vi "Kaelus PIM Config Test.vi"(7 "Str Refnum":refnum<vi>, 8 "error in (no error)":errorcluster, 11 "PIM Configuration":T1={"host IP (localhost)"="localhost", "host Port"=3388, "Model"="", "Serial Number(s)"="", "Calibration Date"=3388.0, "Dual Port?"=FALSE, "DeviceNames"=[], "Parameters"={"TX1start"=0.0, "TX1stop"=0.0, "TX1pmax"=0.0, "TX2start"=0.0, "TX2stop"=0.0, "TX2pmax"=0.0, "RXstart"=0.0, "RXstop"=0.0}, "Interface"=enum."PIM Web Engine"} {"Calibration Date" format="%.2f"; "Parameters"."TX2pmax" format="%.1f"; "Parameters"."TX1pmax" format="%.1f"; "Parameters"."RXstop" format="%.1f"; "Parameters"."RXstart" format="%.1f"; "Parameters"."TX2stop" format="%.1f"; "Parameters"."TX2start" format="%.1f"; "Parameters"."TX1stop" format="%.1f"; "Parameters"."TX1start" format="%.1f"}) -> (0 "error out":errorcluster, 2 "CAL Date (seconds)":dbl, 3 "Serial Number(s)":string)   [LabVIEW 2011]
uses:
  PIM Configuration.ctl
  PIM Interface Language.ctl
  TypeDefs/PIMHW Connection CMDS.ctl
  <userlib>/_OpenG.lib/array/array.llb/Remove Duplicates from 1D Array (String)__ogtk.vi
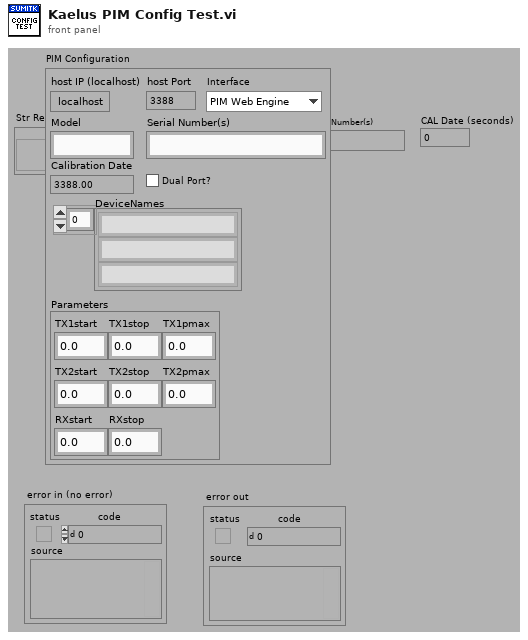
[diagram p1: front panel]
types:
  T1 = typedef "PIM Configuration.ctl" = cluster{"host IP (localhost)":string, "host Port":u16, "Model":string, "Serial Number(s)":string, "Calibration Date":dbl, "Dual Port?":bool, "DeviceNames":string[], "Parameters":cluster{"TX1start":dbl, "TX1stop":dbl, "TX1pmax":dbl, "TX2start":dbl, "TX2stop":dbl, "TX2pmax":dbl, "RXstart":dbl, "RXstop":dbl}, "Interface":T2}
  T2 = typedef "PIM Interface Language.ctl" = enum16{"PIM Web Engine", "PIM HW Engine"}
  T3 = typedef "PIMHW Connection CMDS.ctl" = enum16{"CONNECT", "DISCONNECT", "KEEP_ALIVE"}
  T4 = typedef "Test Set Definition.ctl" = cluster{"General":cluster{"ID":u32, "Model":string, "Dual Port?":bool, "Options String":string, "Options":cluster{"E":bool, "K":bool, "H":bool, "W":bool, "F":bool}, "Cal File":path}, "Receiver":cluster{"Fstart, MHz":dbl, "Fstop MHz":dbl, "Fstep MHz":dbl, "IF, MHz":dbl}, "RX Band":cluster{"Fstart, MHz":dbl, "Fstop MHz":dbl}, "TX 1":cluster{"Fstart, MHz":dbl, "Fstop MHz":dbl, "Pmax, dBm":dbl, "Pstep, dB":dbl}, "TX 2":cluster{"Fstart, MHz":dbl, "Fstop MHz":dbl, "Pmax, dBm":dbl, "Pstep, dB":dbl}, "Low-side?":bool}
  T5 = cluster{"CalVersion":u8, "CalDate":string, "CalSN":string}
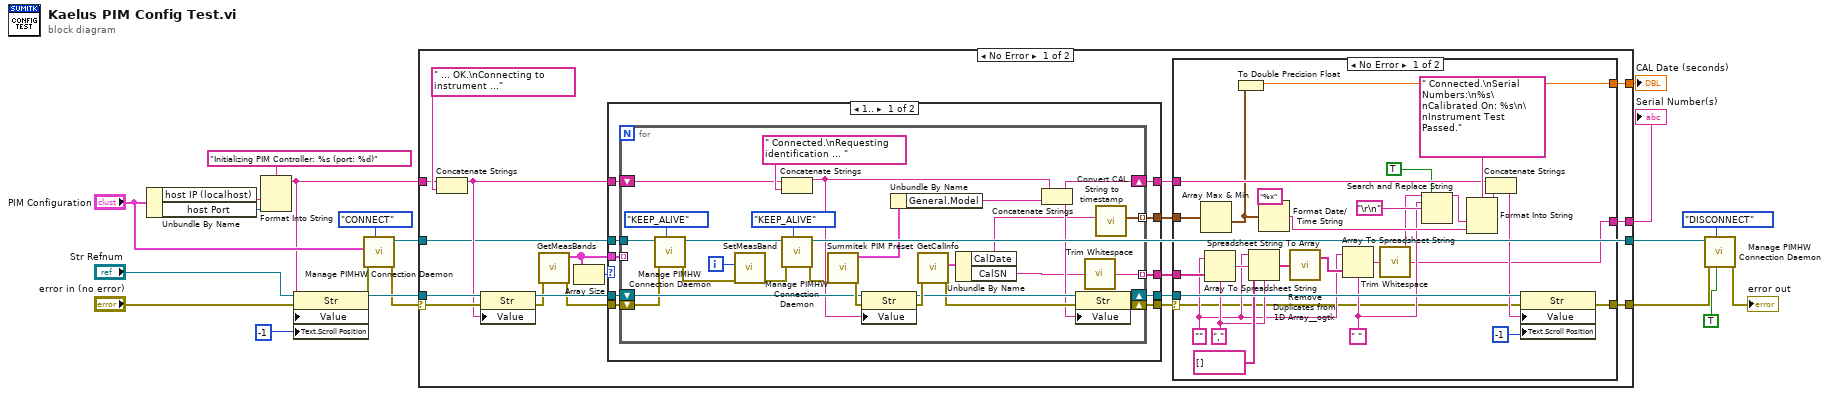
[diagram p0: block diagram]
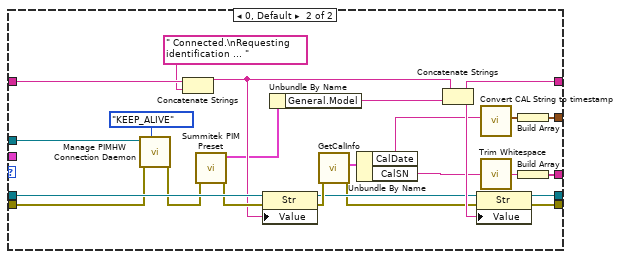
[diagram p2: hidden frame]
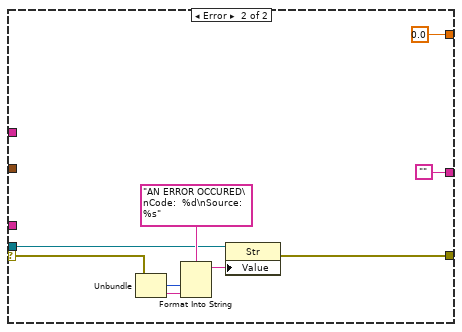
[diagram p3: hidden frame]
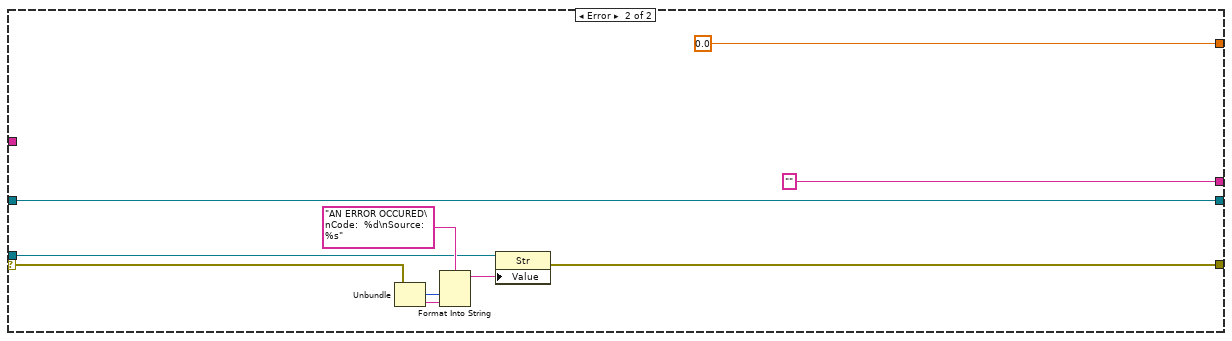
[diagram p4: hidden frame]
diagram:
  n1 = Unbundle By Name("PIM Configuration") -> ("host IP (localhost)"=w19:string, "host Port"=w18:u16)
  n2 = Format Into String(format string="Initializing PIM Controller: %s (port: %d)", w19, w18) -> (resulting string=w12:string)  [unwired: 2 in, 1 out]
  n3 = property class="Str"(reference="Str Refnum", error in="error in (no error)", "Value"=w12, "Text.Scroll Position"=-1) -> (reference out=w11:refnum<vi>, error out=w4:errorcluster)
  n4 = call "Manage PIMHW Connection Daemon.vi"("Session Conn Cmd"=PIMHW_Connection_CMDS."CONNECT", "error in (no error)"=w4, "PIM Config (Connection only)"="PIM Configuration") -> ("error out"=w2:errorcluster, "daemon ref out"=w13:refnum<vi>)  [unwired: 2 in, 5 out]
  n5 = case shown="No Error" w2 {
    selector: w2 -> [w36 w142]
    tunnel: w13 -> [w26 w139]
    tunnel: w12 -> [w38 _]
    tunnel: w11 -> [w37 w141]
    tunnel: [w33 w140] -> w7
    tunnel: [w24 "" ("CalSN")] -> w10
    tunnel: [w26 w139] -> w5
    tunnel: [w27 0.0] -> w1
    frame No Error {
      n6 = Concatenate Strings(w38, " ... OK.\nConnecting to instrument ...") -> (w35:string)
      n7 = property class="Str"(reference=w37, error in=w36, "Value"=w35) -> (reference out=w34:refnum<vi>, error out=w30:errorcluster)
      n8 = call "GetMeasBands.vi"("error in (no error)"=w30) -> ("error out"=w29:errorcluster, "TestSets"=w22:T4[])  [unwired: 1 in, 8 out]
      n9 = Array Size(array=w22) -> (size(s)=w21:i32)
      n10 = case shown="1.." w21 {
        tunnel: w35 -> [w49 w100]
        tunnel: w34 -> [w48 w99]
        tunnel: [w47 w98] -> w32
        tunnel: [w46 w97] -> w31
        tunnel: w29 -> [w45 w81]
        tunnel: w22 -> [w44 _]
        tunnel: [w43 w79] -> w28
        tunnel: w26 -> [w42 w96]
        tunnel: [w41 w78] -> w25
        tunnel: [w40 w95] -> w23
        frame 1.. {
          n11 = for {
            shift-right: [w63] -> w46
            shift-left: w49 -> [w75]
            tunnel: [w56] -> w41 mode=indexing
            shift-right: [w67] -> w40
            shift-left: w45 -> [w53]
            shift-right: [w68] -> w47
            shift-left: w48 -> [w73]
            tunnel: w44 -> [_] mode=indexing
            tunnel: [w60] -> w43 mode=indexing
            tunnel: w42 -> [w51]
            i -> [w62]
            n12 = call "Manage PIMHW Connection Daemon.vi"("Session Conn Cmd"=PIMHW_Connection_CMDS."KEEP_ALIVE", "error in (no error)"=w53, "daemon ref"=w51) -> ("error out"=w52:errorcluster, "daemon ref out"=w50:refnum<vi>)  [unwired: 2 in, 5 out]
            n13 = call "SetMeasBand.vi"("error in (no error)"=w52, "Band Index"=w62) -> ("error out"=w58:errorcluster)  [unwired: 1 in, 8 out]
            n14 = Concatenate Strings(w75, " Connected.\nRequesting identification ... ") -> (w66:string)
            n15 = call "Manage PIMHW Connection Daemon.vi"("Session Conn Cmd"=PIMHW_Connection_CMDS."KEEP_ALIVE", "error in (no error)"=w58, "daemon ref"=w50) -> ("error out"=w57:errorcluster)  [unwired: 2 in, 6 out]
            n16 = call "Summitek PIM Preset.vi"("error in (no error)"=w57) -> ("error out"=w74:errorcluster, "TestSetDef"=w65:T4)  [unwired: 2 in, 7 out]
            n17 = property class="Str"(reference=w73, error in=w74, "Value"=w66) -> (reference out=w70:refnum<vi>, error out=w72:errorcluster)
            n18 = Unbundle By Name(w65) -> ("General.Model"=w64:string)
            n19 = call "GetCalInfo.vi"("error in (no error)"=w72) -> ("error out"=w69:errorcluster, "CalInfo"=w71:T5)  [unwired: 1 in, 8 out]
            n20 = Unbundle By Name(w71) -> ("CalDate"=w61:string, "CalSN"=w55:string)
            n21 = Concatenate Strings(w66, w64) -> (w63:string)
            n22 = property class="Str"(reference=w70, error in=w69, "Value"=w63) -> (reference out=w68:refnum<vi>, error out=w67:errorcluster)
            n23 = call <vilib>:"Trim Whitespace.vi"("string"=w55) -> ("trimmed string"=w56:string)  [unwired: 1 in]
            n24 = call "Convert CAL String to timestamp.vi"("abbreviated date string"=w61) -> ("time stamp"=w60:timestamp)  [unwired: 10 out]
          }
        }
        frame 0, Default {
          n25 = call "Manage PIMHW Connection Daemon.vi"("Session Conn Cmd"=PIMHW_Connection_CMDS."KEEP_ALIVE", "error in (no error)"=w81, "daemon ref"=w96) -> ("error out"=w83:errorcluster)  [unwired: 2 in, 6 out]
          n26 = Concatenate Strings(w100, " Connected.\nRequesting identification ... ") -> (w88:string)
          n27 = call "Summitek PIM Preset.vi"("error in (no error)"=w83) -> ("error out"=w93:errorcluster, "TestSetDef"=w87:T4)  [unwired: 2 in, 7 out]
          n28 = property class="Str"(reference=w99, error in=w93, "Value"=w88) -> (reference out=w90:refnum<vi>, error out=w92:errorcluster)
          n29 = Unbundle By Name(w87) -> ("General.Model"=w86:string)
          n30 = call "GetCalInfo.vi"("error in (no error)"=w92) -> ("error out"=w89:errorcluster, "CalInfo"=w91:T5)  [unwired: 1 in, 8 out]
          n31 = Unbundle By Name(w91) -> ("CalDate"=w85:string, "CalSN"=w82:string)
          n32 = Concatenate Strings(w88, w86) -> (w97:string)
          n33 = property class="Str"(reference=w90, error in=w89, "Value"=w97) -> (reference out=w98:refnum<vi>, error out=w95:errorcluster)
          n34 = call "Convert CAL String to timestamp.vi"("abbreviated date string"=w85) -> ("time stamp"=w80:timestamp)  [unwired: 10 out]
          n35 = call <vilib>:"Trim Whitespace.vi"("string"=w82) -> ("trimmed string"=w77:string)  [unwired: 1 in]
          n36 = Build Array(w80) -> (w79:timestamp[])
          n37 = Build Array(w77) -> (w78:string[])
        }
      }
      n38 = case shown="No Error" w23 {
        selector: w23 -> [w102 w131]
        tunnel: [w126 w130] -> w33
        tunnel: w32 -> [w123 w127]
        tunnel: w31 -> [w122 _]
        tunnel: w28 -> [w117 _]
        tunnel: [w116 0.0] -> w27
        tunnel: w25 -> [w111 _]
        tunnel: [w101 ""] -> w24
        frame No Error {
          w107 = "" ("format string")
          w109 = "," ("delimiter (Tab)")
          w105 = " " ("delimiter (Tab)")
          n39 = Array Max & Min(array=w117) -> (min value=w115:timestamp)  [unwired: 3 out]
          n40 = Array To Spreadsheet String(delimiter (Tab)=w109, array=w111, 3:w107) -> (spreadsheet string=w110:string)
          n41 = To Double Precision Float(number=w115) -> (double precision float=w116:dbl)
          n42 = Spreadsheet String To Array(delimiter (Tab)=w109, format string=w107, spreadsheet string=w110, array type (2D Dbl)=string[] []) -> (array=w108:string[])
          n43 = Format Date/Time String(time format string (%c)="%x", seconds (now)=w115) -> (date/time string=w114:string)  [unwired: 1 out]
          n44 = call-poly <userlib>:"Remove Duplicates from 1D Array__ogtk.vi"("Input Array"=w108) -> ("Output Array"=w118:string[])  [unwired: 1 out]
          n45 = Array To Spreadsheet String(delimiter (Tab)=w105, array=w118, 3:w107) -> (spreadsheet string=w121:string)
          n46 = call <vilib>:"Trim Whitespace.vi"("string"=w121) -> ("trimmed string"=w101:string)  [unwired: 1 in]
          n47 = Search and Replace String(replace all?=TRUE ("replace all? (F)"), input string=w101, search string=w105, replace string="\r\n") -> (result string=w104:string)  [unwired: 1 in, 6 out]
          n48 = Format Into String(format string=" Connected.\nSerial Numbers:\n%s\nCalibrated On: %s\n\nInstrument Test Passed.", w104, w114) -> (resulting string=w124:string)  [unwired: 2 in, 1 out]
          n49 = Concatenate Strings(w122, w124) -> (w120:string)
          n50 = property class="Str"(reference=w123, error in=w102, "Value"=w120, "Text.Scroll Position"=-1) -> (error out=w126:errorcluster)  [unwired: 1 out]
        }
        frame Error {
          n51 = Unbundle(w131) -> ("code"=w133:i32, "source"=w132:string)  [unwired: 1 out]
          n52 = Format Into String(format string="AN ERROR OCCURED\nCode:  %d\nSource: %s", w133, w132) -> (resulting string=w135:string)  [unwired: 2 in, 1 out]
          n53 = property class="Str"(reference=w127, "Value"=w135) -> (error out=w130:errorcluster)  [unwired: 1 in, 1 out]
        }
      }
    }
    frame Error {
      n54 = Unbundle(w142) -> ("code"=w144:i32, "source"=w145:string)  [unwired: 1 out]
      n55 = Format Into String(format string="AN ERROR OCCURED\nCode:  %d\nSource: %s", w144, w145) -> (resulting string=w137:string)  [unwired: 2 in, 1 out]
      n56 = property class="Str"(reference=w141, "Value"=w137) -> (error out=w140:errorcluster)  [unwired: 1 in, 1 out]
    }
  }
  "Serial Number(s)" <- w10
  "CAL Date (seconds)" <- w1
  n57 = call "Manage PIMHW Connection Daemon.vi"("Disconnect TCP? (f)"=TRUE, "Session Conn Cmd"=PIMHW_Connection_CMDS."DISCONNECT", "error in (no error)"=w7, "daemon ref"=w5) -> ("error out"=→"error out":errorcluster)  [unwired: 1 in, 6 out]
